vi "main.vi"() -> ()   [LabVIEW 2020]
uses:
  <vilib>/express/express arith-compare/Formula/XNode/ExpressFormulaBlockNode.xnode
  <vilib>/measure/NI_MABase.lvlib
panel:
  in  "?":enum32{"单个取样值", "连续的模拟信号", "自定义非均匀量化"}(tab)
  in  "量化阶 V 2":dbl=0.02
  out "数字编码":dbl[](array[numeric])
  in  "输入的模拟信号取样值 V":dbl(ring)=0.075 items=["0.075"=0.075, "0.130"=0.13, "0.131"=0.131, "1.239"=1.239, "2.510"=2.51, "-2.540"=-2.54, "-2.700"=-2.7]
  out "复原的模拟信号 V":dbl
  out "量化误差 V":dbl
  out "瞬时量化信噪比 dB":dbl
  out "瞬时量化信噪比 dB":dbl
  out "量化误差 V":dbl
  out "复原的模拟信号 V":dbl
  out "数字编码":dbl[](array[numeric])
  in  "Vref V":dbl=2.56
  in  "A V":dbl(ring)=2.5 items=["2.5"=2.5, "0.64"=0.64, "0.1"=0.1, "3"=3.0]
  in  "f Hz":dbl=100.0
  in  "量化阶 V":dbl=0.02
  in  "仿真过采样率":dbl=1000.0
  out "输入模拟信号波形":waveform(dbl)(graph)
  out "复原的模拟信号波形":waveform(dbl)(graph)
  out "量化噪声波形":waveform(dbl)(graph)
  out "量化信噪比 dB":dbl
  out "理论量化信噪比 dB":dbl
  out "量化信噪比 dB":dbl
  out "量化噪声波形":waveform(dbl)(graph)
  out "复原的模拟信号波形":waveform(dbl)(graph)
  in  "Vref V":dbl=2.56
  out "量化信噪比 dB":dbl
  in  "Vref V":dbl=2.56
  out "量化信噪比 dB":dbl
  in  "量化阶 V 3":dbl=0.02
  out "量化信噪比 dB":dbl
  in  "Vref V":dbl=2.56
  out "13折线量化噪声波形":dbl[](graph)
  out "均匀量化噪声波形":dbl[](graph)
  out "自定义非均匀量化噪声波形":dbl[](graph)
  out "fs Hz":dbl
  # "均匀量化"
  # "非均匀量化"
  # "输入参数"
  # "均匀量化"
  # "非均匀量化"
  # "均匀量化"
  # "13折线量化"
  # "自定义非均匀量化"
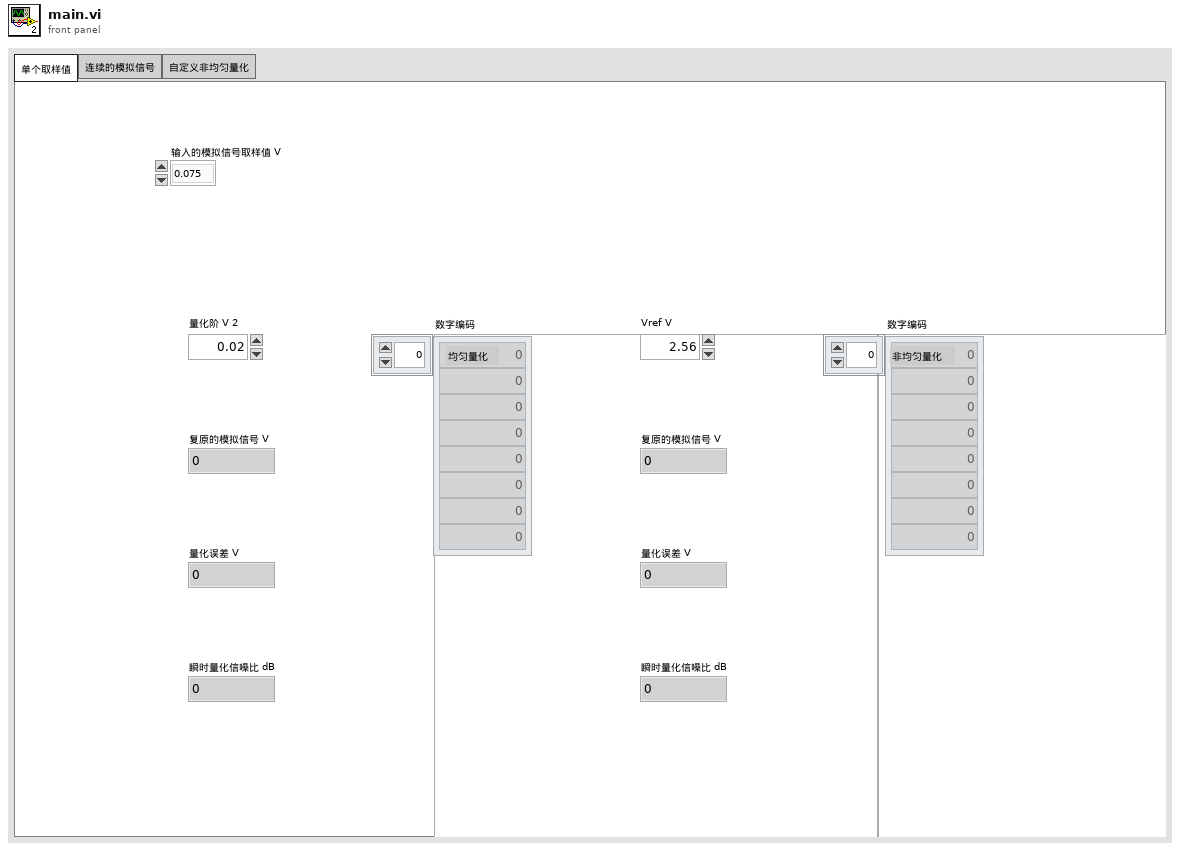
[diagram p1: front panel]
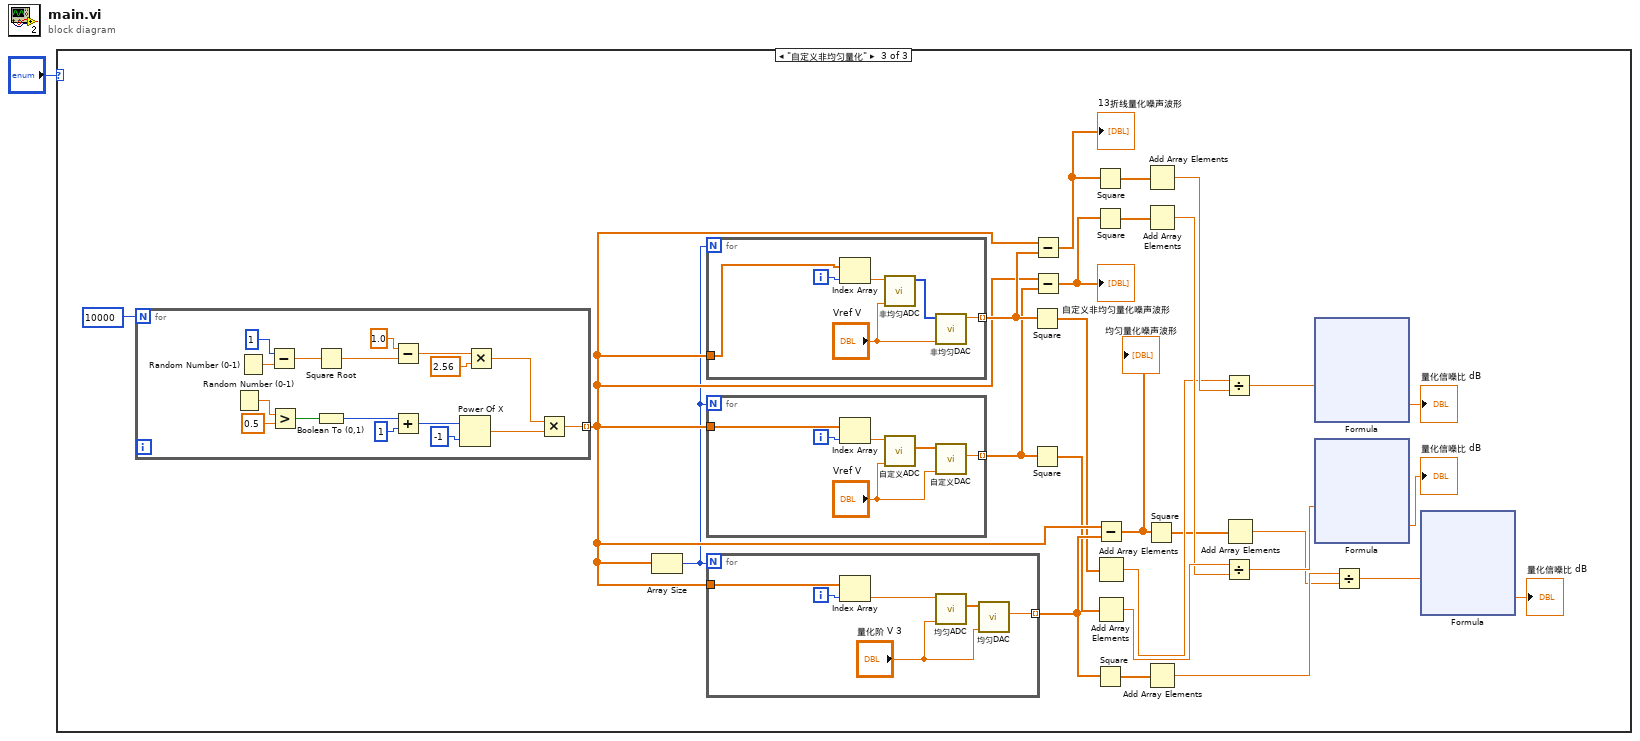
[diagram p0: block diagram]
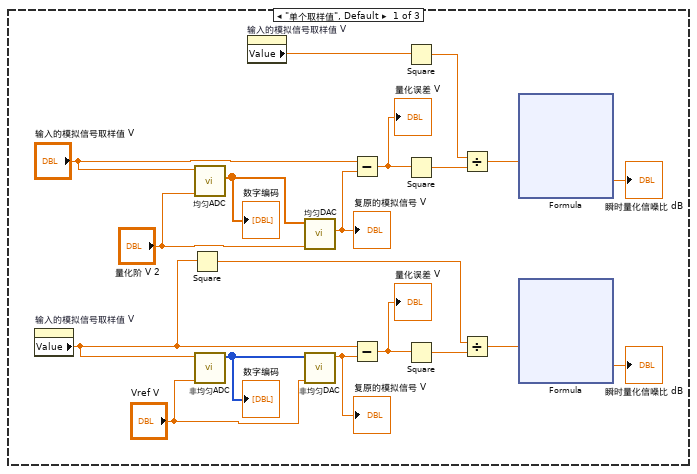
[diagram p2: hidden frame]
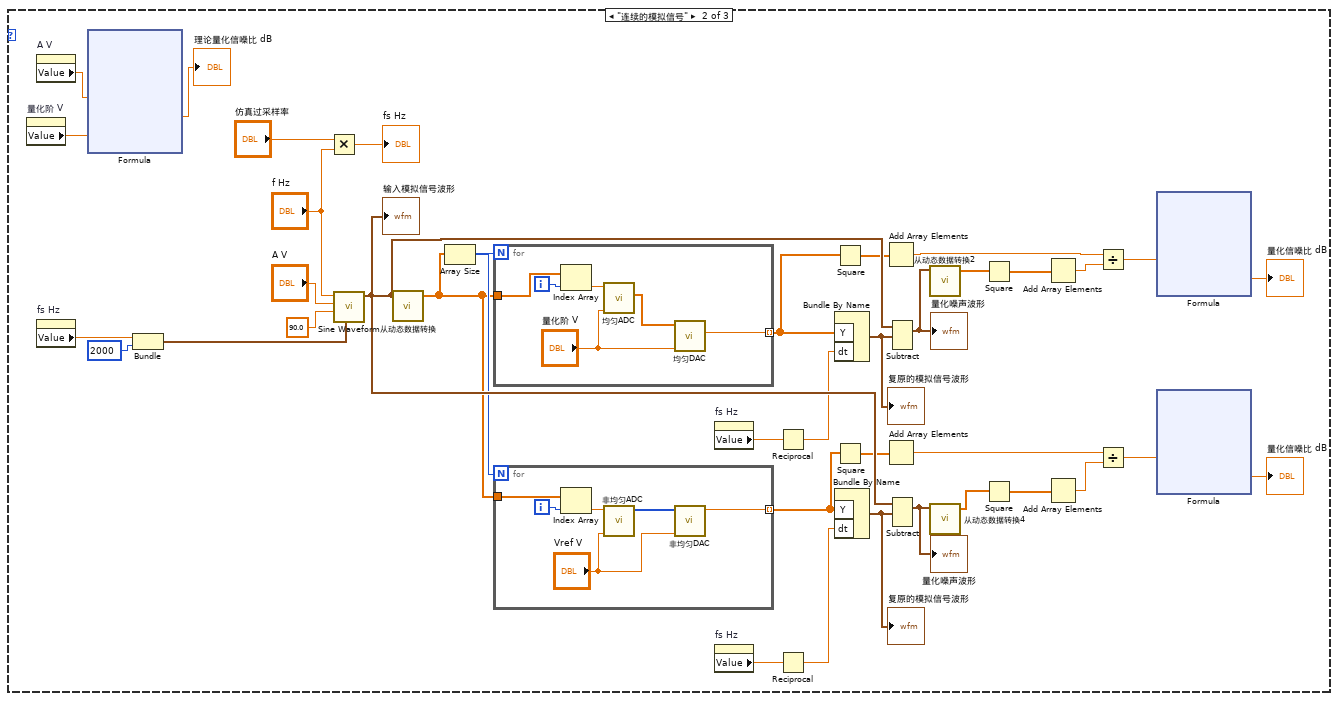
[diagram p3: hidden frame]
diagram:
  n1 = case shown="\"自定义非均匀量化\"" "?" {
    frame "单个取样值", Default {
      n2 = property on="输入的模拟信号取样值 V" class="Ring (strict)"() -> ("Value"=w20:dbl)  [unwired: 2 in, 2 out]
      n3 = Square(x=w20) -> (x^2=w11:dbl)
      n4 = call "均匀ADC.vi"("量化阶 V"="量化阶 V 2", "输入的模拟信号取样值 V"="输入的模拟信号取样值 V") -> ("数字编码"=w2:dbl[])  [unwired: 9 in]
      "数字编码" <- w2
      n5 = call "非均匀ADC.vi"("输入的模拟信号取样值 V"=w20, "Vref V"="Vref V") -> ("数字编码"=w19:i32[])  [unwired: 8 in]
      "数字编码" <- w19
      n6 = property on="输入的模拟信号取样值 V" class="Ring (strict)"() -> ("Value"=w5:dbl)  [unwired: 2 in, 2 out]
      n7 = call "均匀DAC.vi"("量化阶 V"="量化阶 V 2", "数字编码"=w2) -> ("x+y"=w4:dbl)  [unwired: 9 in]
      "复原的模拟信号 V" <- w4
      n8 = call "非均匀DAC.vi"("Vref V"="Vref V", "数字编码"=w19) -> ("x+y 2"=w12:dbl)  [unwired: 9 in]
      "复原的模拟信号 V" <- w12
      n9 = Subtract(x="输入的模拟信号取样值 V", y=w4) -> (x-y=w10:dbl)
      "量化误差 V" <- w10
      n10 = Subtract(x=w20, y=w12) -> (x-y=w16:dbl)
      "量化误差 V" <- w16
      n11 = Square(x=w5) -> (x^2=w6:dbl)
      n12 = Square(x=w10) -> (x^2=w7:dbl)
      n13 = Square(x=w16) -> (x^2=w13:dbl)
      n14 = Divide(x=w6, y=w7) -> (x/y=w8:dbl)
      n15 = Divide(x=w11, y=w13) -> (x/y=w14:dbl)
      n16 = xnode "Formula"("X1"=w8) -> ("Result"=→"瞬时量化信噪比 dB":dbl)  [unwired: 1 in, 1 out]
      n17 = xnode "Formula"("X1"=w14) -> ("Result"=→"瞬时量化信噪比 dB":dbl)  [unwired: 1 in, 1 out]
    }
    frame "连续的模拟信号" {
      n18 = property on="量化阶 V" class="DigNum (strict)"() -> ("Value"=w38:dbl)  [unwired: 2 in, 2 out]
      n19 = property on="A V" class="Ring (strict)"() -> ("Value"=w37:dbl)  [unwired: 2 in, 2 out]
      n20 = property on="fs Hz" class="DigNum (strict)"() -> ("Value"=w46:dbl)  [unwired: 2 in, 2 out]
      n21 = xnode "Formula"("A"=w37, "delta"=w38) -> ("Result"=→"理论量化信噪比 dB":dbl)  [unwired: 1 in, 1 out]
      n22 = Bundle("Value"=w46, 2000) -> (w47:cluster{"Value":dbl, i32})  [unwired: 1 in]
      n23 = Multiply(x="仿真过采样率", y="f Hz") -> (x*y=→"fs Hz":dbl)
      n24 = call <vilib>:"Sine Waveform.vi"("sampling info"=w47, "phase"=90.0, "amplitude"="A V", "frequency"="f Hz") -> ("signal out"=w74:waveform(dbl))  [unwired: 6 in, 1 out]
      "输入模拟信号波形" <- w74
      n25 = call "从动态数据转换"("Dynamic Data Type"=w74) -> ("Array"=w72:dbl[])  [unwired: 3 in]
      n26 = Array Size(array=w72) -> (size(s)=w73:i32)
      n27 = for {
        N: w73 -> [_]
        tunnel: w72 -> [w110]
        tunnel: [w107] -> w51 mode=indexing
        i -> [w112]
        n28 = Index Array(array=w110, index=w112) -> (element=w111:dbl)
        n29 = call "均匀ADC.vi"("量化阶 V"="量化阶 V", "输入的模拟信号取样值 V"=w111) -> ("数字编码"=w109:dbl[])  [unwired: 9 in]
        n30 = call "均匀DAC.vi"("量化阶 V"="量化阶 V", "数字编码"=w109) -> ("x+y"=w107:dbl)  [unwired: 9 in]
      }
      n31 = for {
        N: w73 -> [_]
        tunnel: w72 -> [w97]
        tunnel: [w96] -> w68 mode=indexing
        i -> [w98]
        n32 = Index Array(array=w97, index=w98) -> (element=w95:dbl)
        n33 = call "非均匀ADC.vi"("输入的模拟信号取样值 V"=w95, "Vref V"="Vref V") -> ("数字编码"=w93:i32[])  [unwired: 8 in]
        n34 = call "非均匀DAC.vi"("Vref V"="Vref V", "数字编码"=w93) -> ("x+y 2"=w96:dbl)  [unwired: 9 in]
      }
      n35 = property on="fs Hz" class="DigNum (strict)"() -> ("Value"=w48:dbl)  [unwired: 2 in, 2 out]
      n36 = property on="fs Hz" class="DigNum (strict)"() -> ("Value"=w71:dbl)  [unwired: 2 in, 2 out]
      n37 = Reciprocal(x=w48) -> (1/x=w49:dbl)
      n38 = Reciprocal(x=w71) -> (1/x=w70:dbl)
      n39 = Square(x=w51) -> (x^2=w52:dbl[])
      n40 = Bundle By Name("Y"=w51, "dt"=w49) -> (w50:waveform(dbl))  [unwired: 1 in]
      "复原的模拟信号波形" <- w50
      n41 = Square(x=w68) -> (x^2=w67:dbl[])
      n42 = Bundle By Name("Y"=w68, "dt"=w70) -> (w69:waveform(dbl))  [unwired: 1 in]
      "复原的模拟信号波形" <- w69
      n43 = Add Array Elements(numeric array=w52) -> (sum=w57:dbl)
      n44 = Add Array Elements(numeric array=w67) -> (sum=w62:dbl)
      n45 = Subtract(1:w50, 2:w74) -> (0:w54:waveform(dbl))  [unwired: 1 in, 1 out]
      "量化噪声波形" <- w54
      n46 = Subtract(1:w69, 2:w74) -> (0:w65:waveform(dbl))  [unwired: 1 in, 1 out]
      "量化噪声波形" <- w65
      n47 = call "从动态数据转换2"("Dynamic Data Type"=w54) -> ("Array"=w55:dbl[])  [unwired: 3 in]
      n48 = call "从动态数据转换4"("Dynamic Data Type"=w65) -> ("Array"=w64:dbl[])  [unwired: 3 in]
      n49 = Square(x=w55) -> (x^2=w53:dbl[])
      n50 = Square(x=w64) -> (x^2=w66:dbl[])
      n51 = Add Array Elements(numeric array=w53) -> (sum=w56:dbl)
      n52 = Add Array Elements(numeric array=w66) -> (sum=w63:dbl)
      n53 = Divide(x=w57, y=w56) -> (x/y=w59:dbl)
      n54 = Divide(x=w62, y=w63) -> (x/y=w60:dbl)
      n55 = xnode "Formula"("X1"=w59) -> ("Result"=→"量化信噪比 dB":dbl)  [unwired: 1 in, 1 out]
      n56 = xnode "Formula"("X1"=w60) -> ("Result"=→"量化信噪比 dB":dbl)  [unwired: 1 in, 1 out]
    }
    frame "自定义非均匀量化" {
      n57 = for {
        N: 10000 -> [_]
        tunnel: [w140] -> w133 mode=indexing
        n58 = Random Number (0-1)() -> (number: 0 to 1=w155:dbl)
        n59 = Random Number (0-1)() -> (number: 0 to 1=w147:dbl)
        n60 = Subtract(x=1, y=w147) -> (x-y=w146:dbl)
        n61 = Greater?(x=w155, y=0.5) -> (0:w150:bool)
        n62 = Square Root(x=w146) -> (sqrt(x)=w144:dbl)
        n63 = Boolean To (0,1)(Boolean=w150) -> (0, 1=w149:i16)
        n64 = Subtract(x=1.0 ("y"), y=w144) -> (x-y=w143:dbl)
        n65 = Add(x=w149, y=1) -> (x+y=w153:i32)
        n66 = Power Of X(1:-1 ("x"), 2:w153) -> (0:w141:dbl)
        n67 = Multiply(x=w143, y=2.56) -> (x*y=w142:dbl)
        n68 = Multiply(x=w142, y=w141) -> (x*y=w140:dbl)
      }
      n69 = Array Size(array=w133) -> (size(s)=w132:i32)
      n70 = for {
        N: w132 -> [_]
        tunnel: w133 -> [w183]
        tunnel: [w182] -> w136 mode=indexing
        i -> [w184]
        n71 = Index Array(array=w183, index=w184) -> (element=w181:dbl)
        n72 = call "非均匀ADC.vi"("输入的模拟信号取样值 V"=w181, "Vref V"="Vref V") -> ("数字编码"=w179:i32[])  [unwired: 8 in]
        n73 = call "非均匀DAC.vi"("Vref V"="Vref V", "数字编码"=w179) -> ("x+y 2"=w182:dbl)  [unwired: 9 in]
      }
      n74 = for {
        N: w132 -> [_]
        tunnel: [w165] -> w134 mode=indexing
        tunnel: w133 -> [w169]
        i -> [w170]
        n75 = Index Array(array=w169, index=w170) -> (element=w167:dbl)
        n76 = call "自定义ADC.vi"("Vref V"="Vref V", "输入 V"=w167) -> ("数字编码"=w168:dbl[])  [unwired: 9 in]
        n77 = call "自定义DAC.vi"("Vref V"="Vref V", "数字编码"=w168) -> ("输出 V"=w165:dbl)  [unwired: 9 in]
      }
      n78 = for {
        N: w132 -> [_]
        tunnel: w133 -> [w196]
        tunnel: [w193] -> w138 mode=indexing
        i -> [w198]
        n79 = Index Array(array=w196, index=w198) -> (element=w197:dbl)
        n80 = call "均匀ADC.vi"("量化阶 V"="量化阶 V 3", "输入的模拟信号取样值 V"=w197) -> ("数字编码"=w195:dbl[])  [unwired: 9 in]
        n81 = call "均匀DAC.vi"("量化阶 V"="量化阶 V 3", "数字编码"=w195) -> ("x+y"=w193:dbl)  [unwired: 9 in]
      }
      n82 = Square(x=w136) -> (x^2=w125:dbl[])
      n83 = Square(x=w134) -> (x^2=w126:dbl[])
      n84 = Subtract(x=w133, y=w136) -> (x-y=w137:dbl[])
      "13折线量化噪声波形" <- w137
      n85 = Subtract(x=w133, y=w134) -> (x-y=w135:dbl[])
      "自定义非均匀量化噪声波形" <- w135
      n86 = Square(x=w137) -> (x^2=w124:dbl[])
      n87 = Square(x=w135) -> (x^2=w127:dbl[])
      n88 = Square(x=w138) -> (x^2=w114:dbl[])
      n89 = Subtract(x=w133, y=w138) -> (x-y=w139:dbl[])
      "均匀量化噪声波形" <- w139
      n90 = Add Array Elements(numeric array=w125) -> (sum=w122:dbl)
      n91 = Add Array Elements(numeric array=w126) -> (sum=w129:dbl)
      n92 = Square(x=w139) -> (x^2=w115:dbl[])
      n93 = Add Array Elements(numeric array=w124) -> (sum=w123:dbl)
      n94 = Add Array Elements(numeric array=w127) -> (sum=w128:dbl)
      n95 = Add Array Elements(numeric array=w114) -> (sum=w117:dbl)
      n96 = Divide(x=w122, y=w123) -> (x/y=w120:dbl)
      n97 = Divide(x=w129, y=w128) -> (x/y=w131:dbl)
      n98 = Add Array Elements(numeric array=w115) -> (sum=w116:dbl)
      n99 = xnode "Formula"("X1"=w120) -> ("Result"=→"量化信噪比 dB":dbl)  [unwired: 1 in, 1 out]
      n100 = xnode "Formula"("X1"=w131) -> ("Result"=→"量化信噪比 dB":dbl)  [unwired: 1 in, 1 out]
      n101 = Divide(x=w117, y=w116) -> (x/y=w119:dbl)
      n102 = xnode "Formula"("X1"=w119) -> ("Result"=→"量化信噪比 dB":dbl)  [unwired: 1 in, 1 out]
    }
  }
